vi "HEWH Filter Bad Data_Sub1.vi"(4 "Data":i32=22, 8 "error in (no error)":errorcluster, 10 "Full DBL Array":dbl[][](array[numeric]), 11 "Full String Array":string[][](array[string])) -> (0 "error out":errorcluster, 1 "Message String":string, 2 "Full DBL Array Out":dbl[][](array[numeric]), 3 "Full String Array Out":string[][](array[string]))   [LabVIEW 2023]
panel:
  out "subarray":string[](array[string])
  out "Array":string[](array[string])
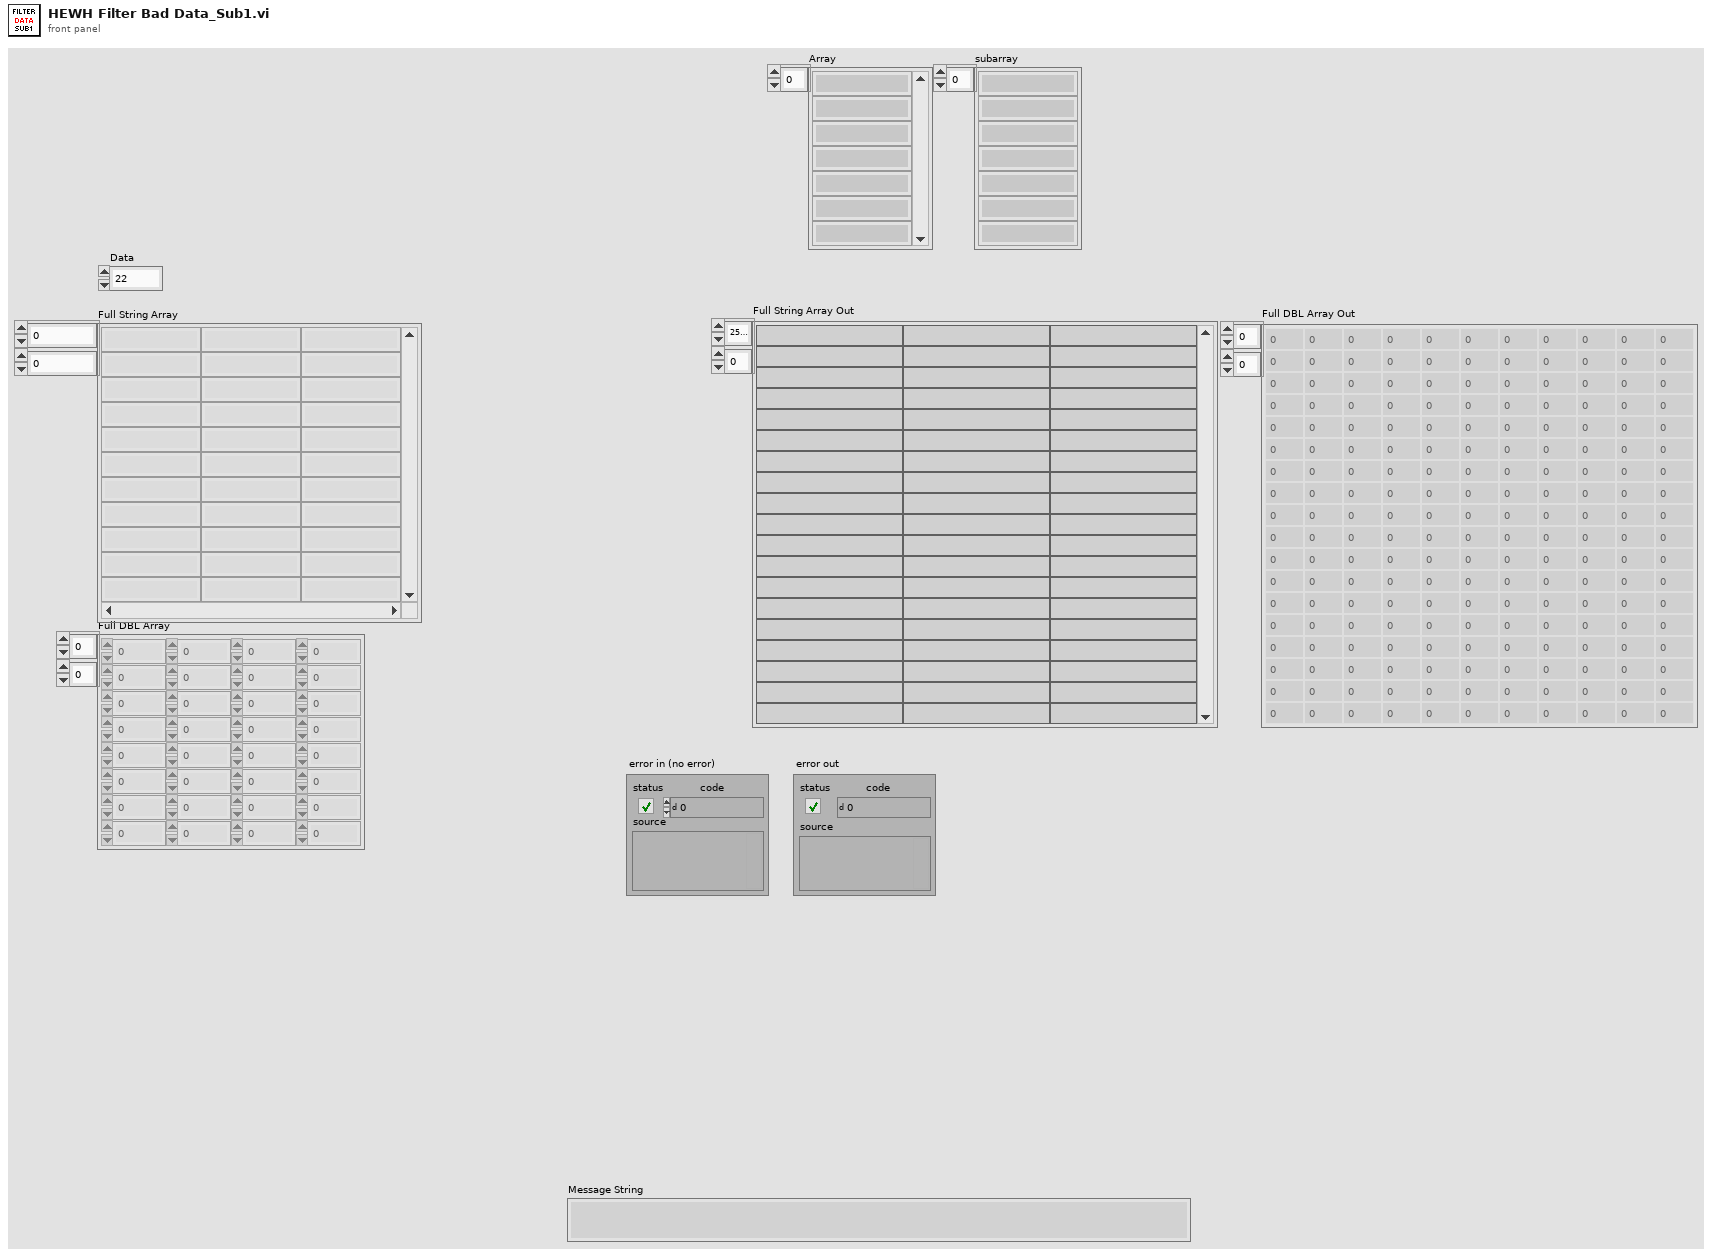
[diagram p1: front panel]
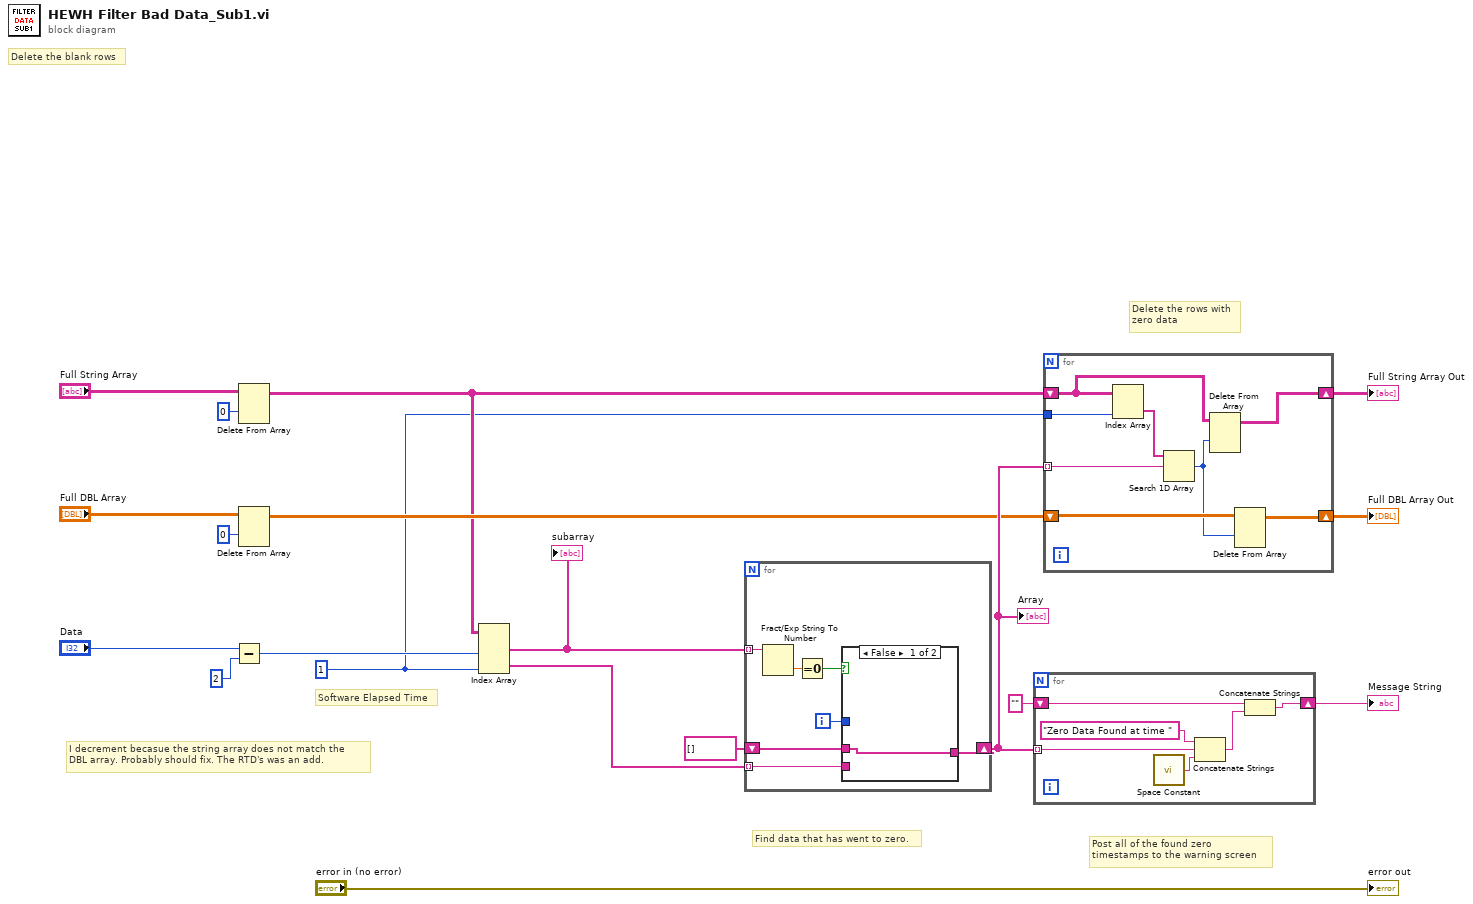
[diagram p0: block diagram]
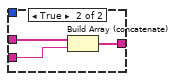
[diagram p2: hidden frame]
diagram:
  w1 = 1 ("Timestamp")
  # "I decrement becasue the string array does not match the \nDBL array. Probably should fix. The RTD's was an add."
  # "Delete the blank rows"
  # "Post all of the found zero \ntimestamps to the warning screen"
  # "Software Elapsed Time"
  # "Delete the rows with\nzero data"
  # "Find data that has went to zero."
  n1 = Subtract(x="Data", y=2) -> (x-y=w8:i32)
  n2 = Delete From Array(array="Full String Array", index (row)=0) -> (array with subset deleted=w2:string[][])  [unwired: 2 in, 1 out]
  n3 = Delete From Array(array="Full DBL Array", index (row)=0) -> (array with subset deleted=w3:dbl[][])  [unwired: 2 in, 1 out]
  n4 = Index Array(array=w2, index (col) #1=w8, index (col) #2=w1) -> (element #1=w12:string[], element #2=w11:string[])  [unwired: 2 in]
  "subarray" <- w12
  n5 = for {
    tunnel: w12 -> [w26] mode=indexing
    shift-right: [w22] -> w17
    shift-left: string[] [] -> [w23]
    tunnel: w11 -> [w21] mode=indexing
    i -> [w20]
    n6 = Fract/Exp String To Number(string=w26) -> (number=w25:dbl)  [unwired: 3 in, 1 out]
    n7 = Equal To 0?(x=w25) -> (x = 0?=w24:bool)
    n8 = case shown="False" w24 {
      tunnel: w20 -> [_ _]
      tunnel: w23 -> [w27 w30]
      tunnel: [w27 w29] -> w22
      tunnel: w21 -> [_ w28]
      frame False {
      }
      frame True {
        n9 = Build Array (concatenate)(w30, w28) -> (w29:string[])
      }
    }
  }
  "Array" <- w17
  n10 = for {
    tunnel: w17 -> [w36] mode=indexing
    shift-right: [w32] -> w19
    shift-left: "" ("string") -> [w33]
    n11 = call <vilib>:"Space Constant.vi"() -> ("String"=w31:string)
    n12 = Concatenate Strings("Zero Data Found at time " ("string"), w36, w31) -> (w34:string)
    n13 = Concatenate Strings(w33, w34) -> (w32:string)
  }
  "Message String" <- w19
  n14 = for {
    tunnel: w17 -> [w44] mode=indexing
    shift-right: [w41] -> w15
    shift-left: w2 -> [w42]
    shift-right: [w38] -> w16
    shift-left: w3 -> [w40]
    tunnel: w1 -> [w37]
    n15 = Index Array(array=w42, index (col)=w37) -> (element=w43:string[])  [unwired: 1 in]
    n16 = Search 1D Array(1D array=w43, element=w44) -> (index of element=w39:i32)  [unwired: 1 in]
    n17 = Delete From Array(array=w42, index (row)=w39) -> (array with subset deleted=w41:string[][])  [unwired: 2 in, 1 out]
    n18 = Delete From Array(array=w40, index (row)=w39) -> (array with subset deleted=w38:dbl[][])  [unwired: 2 in, 1 out]
  }
  "Full String Array Out" <- w15
  "Full DBL Array Out" <- w16
  "error out" <- "error in (no error)"
